vi "subFilterResultsTopLevel.vi"(8 "error in (no error)":errorcluster, 11 "CDependencyInspection in":refnum<class "CDependencyInspection.lvclass">) -> (0 "error out":errorcluster, 3 "CDependencyInspection out":refnum<class "CDependencyInspection.lvclass">)   [LabVIEW 2020, in "DependencyInspection.lvlib" / "CDependencyInspection.lvclass"]
uses:
  CDependencyInspection.lvclass
  CDependencyInspection.lvclass/CDependencyInspection.ctl
  CDependencyList/CDependencyList.lvclass
  obj/Addons/LabVIEWObjectInterfaces.lvlibp/LabVIEWObjectInterfaces/ILabVIEWItem/ILabVIEWItem.lvclass
  obj/Addons/LabVIEWObjectFactory.lvlibp
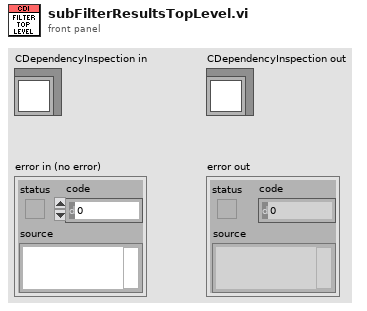
[diagram p1: front panel]
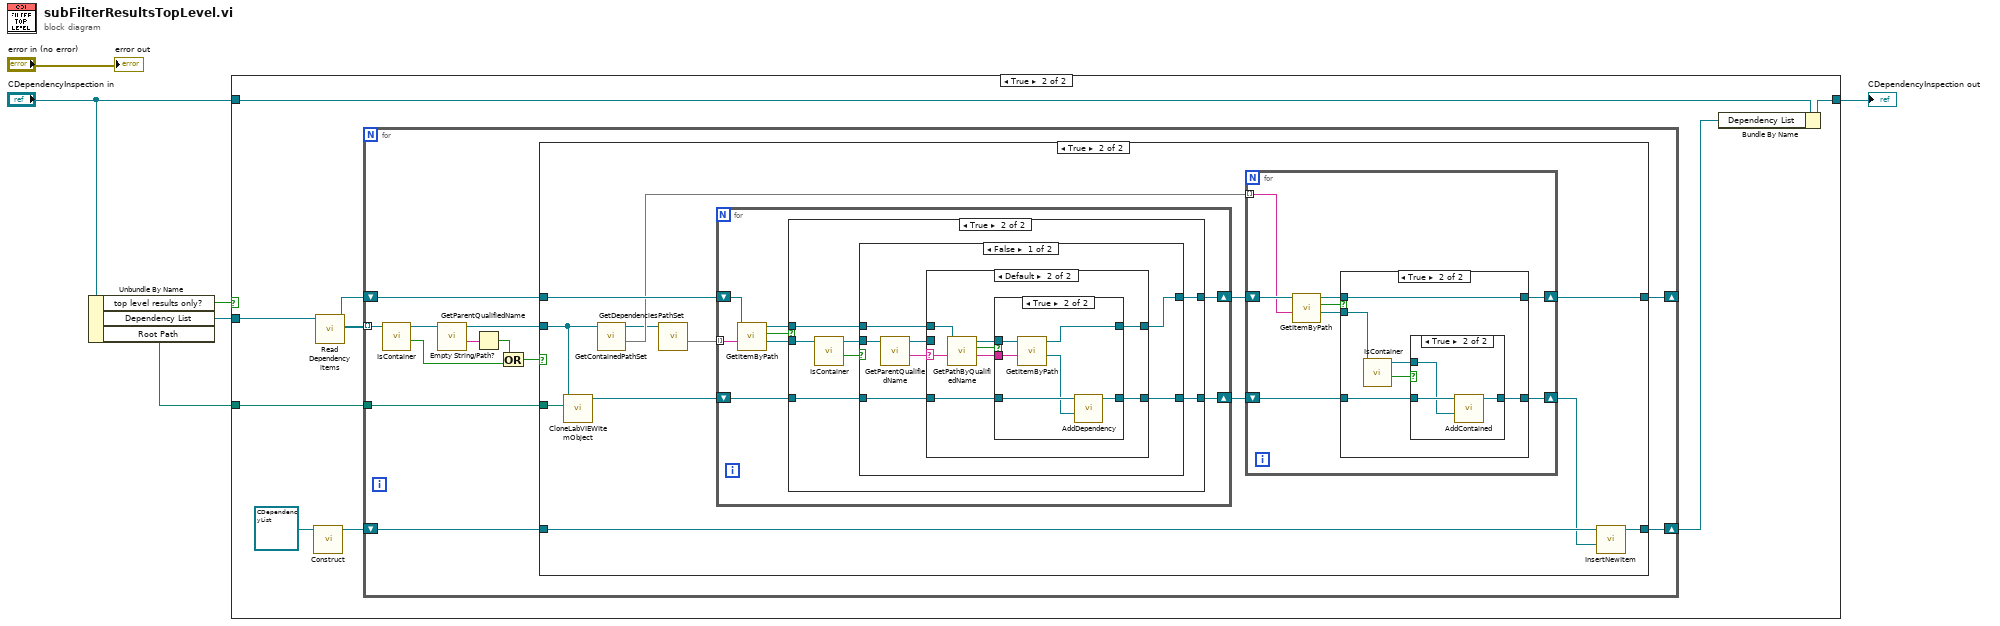
[diagram p0: block diagram]
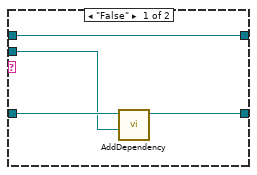
[diagram p5: hidden frame]
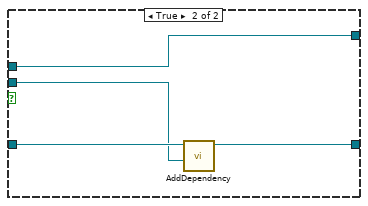
[diagram p7: hidden frame]
diagram:
  n1 = Unbundle By Name("CDependencyInspection in") -> ("top level results only?"=w3:bool, "Dependency List"=w5:refnum<class "CDependencyList.lvclass">, "Root Path"=w4:path)
  n2 = case shown="True" w3 {
    tunnel: w5 -> [_ w13]
    tunnel: w4 -> [_ w12]
    tunnel: "CDependencyInspection in" -> [w7 w10]
    tunnel: [w7 w9] -> w1
    frame False {
    }
    frame True {
      n3 = call-dynamic "Construct.vi"("CDependencyList in"=refnum<class "CDependencyList.lvclass"> refnum) -> ("CDependencyList out"=w11:refnum<class "CDependencyList.lvclass">)  [unwired: 9 in, 1 out]
      n4 = call-dynamic "Read Dependency items.vi"("CDependencyList in"=w13) -> ("Dependency items"=w16:refnum<class "ILabVIEWItem.lvclass">[], "CDependencyList out"=w14:refnum<class "CDependencyList.lvclass">)  [unwired: 9 in]
      n5 = for {
        tunnel: w16 -> [w28] mode=indexing
        shift-right: [w25] -> _
        shift-left: w14 -> [w26]
        tunnel: w12 -> [w27]
        shift-right: [w23] -> w8
        shift-left: w11 -> [w24]
        n6 = call-dynamic "IsContainer.vi"("ILabVIEWItem in"=w28) -> ("Is container?"=w18:bool, "ILabVIEWItem out"=w22:refnum<class "ILabVIEWItem.lvclass">)  [unwired: 8 in, 1 out]
        n7 = call-dynamic "GetParentQualifiedName.vi"("ILabVIEWItem in"=w22) -> ("Name"=w20:string, "ILabVIEWItem out"=w21:refnum<class "ILabVIEWItem.lvclass">)  [unwired: 8 in, 1 out]
        n8 = Empty String/Path?(string/path=w20) -> (empty?=w19:bool)
        n9 = Or(x=w19, y=w18) -> (x .or. y?=w17:bool)
        n10 = case shown="True" w17 {
          tunnel: w27 -> [_ w42]
          tunnel: w26 -> [w30 w40]
          tunnel: [w30 w38] -> w25
          tunnel: w24 -> [w29 w36]
          tunnel: [w29 w34] -> w23
          tunnel: w21 -> [_ w32]
          frame False {
          }
          frame True {
            n11 = call "CloneLabVIEWItemObject.vi"("Root path"=w42, "ILabVIEWItem in"=w32) -> ("Cloned ILabVIEWItem"=w41:refnum<class "ILabVIEWItem.lvclass">)  [unwired: 9 in]
            n12 = call-dynamic "GetContainedPathSet.vi"("ILabVIEWItem in"=w32) -> ("Contained"=w33:set{string}, "ILabVIEWItem out"=w31:refnum<class "ILabVIEWItem.lvclass">)  [unwired: 8 in, 1 out]
            n13 = call-dynamic "GetDependenciesPathSet.vi"("ILabVIEWItem in"=w31) -> ("Dependencies"=w43:set{string})  [unwired: 8 in, 2 out]
            n14 = for {
              tunnel: w43 -> [w51] mode=indexing
              shift-right: [w47] -> w37
              shift-left: w41 -> [w48]
              shift-right: [w44] -> w39
              shift-left: w40 -> [w46]
              n15 = call-dynamic "GetItemByPath.vi"("Path"=w51, "CDependencyList in"=w46) -> ("ILabVIEWItem"=w49:refnum<class "ILabVIEWItem.lvclass">, "key found?"=w50:bool, "CDependencyList out"=w45:refnum<class "CDependencyList.lvclass">)  [unwired: 6 in, 1 out]
              n16 = case shown="True" w50 {
                tunnel: w49 -> [_ w60]
                tunnel: w48 -> [w53 w58]
                tunnel: [w53 w56] -> w47
                tunnel: w45 -> [w52 w55]
                tunnel: [w52 w54] -> w44
                frame False {
                }
                frame True {
                  n17 = call-dynamic "IsContainer.vi"("ILabVIEWItem in"=w60) -> ("Is container?"=w59:bool, "ILabVIEWItem out"=w57:refnum<class "ILabVIEWItem.lvclass">)  [unwired: 8 in, 1 out]
                  n18 = case shown="False" w59 {
                    tunnel: w58 -> [w65 w91]
                    tunnel: w57 -> [w67 w90]
                    tunnel: [w63 w89] -> w56
                    tunnel: w55 -> [w66 w88]
                    tunnel: [w64 w88] -> w54
                    frame False {
                      n19 = call-dynamic "GetParentQualifiedName.vi"("ILabVIEWItem in"=w67) -> ("Name"=w62:string, "ILabVIEWItem out"=w61:refnum<class "ILabVIEWItem.lvclass">)  [unwired: 8 in, 1 out]
                      n20 = case shown="Default" w62 {
                        selector: w62 -> [_ w72]
                        tunnel: w66 -> [w68 w79]
                        tunnel: w65 -> [w71 w75]
                        tunnel: [w68 w74] -> w64
                        tunnel: [w70 w73] -> w63
                        tunnel: w61 -> [w69 _]
                        frame "False" {
                          n21 = call-dynamic "AddDependency.vi"("Item to depend on"=w69, "ILabVIEWItem in"=w71) -> ("ILabVIEWItem out"=w70:refnum<class "ILabVIEWItem.lvclass">)  [unwired: 8 in, 1 out]
                        }
                        frame Default {
                          n22 = call-dynamic "GetPathByQualifiedName.vi"("Qualified name"=w72, "CDependencyList in"=w79) -> ("Path"=w77:string, "key found?"=w78:bool, "CDependencyList out"=w76:refnum<class "CDependencyList.lvclass">)  [unwired: 6 in, 1 out]
                          n23 = case shown="True" w78 {
                            tunnel: w77 -> [_ w86]
                            tunnel: w76 -> [w81 w87]
                            tunnel: w75 -> [w80 w85]
                            tunnel: [w81 w83] -> w74
                            tunnel: [w80 w82] -> w73
                            frame False {
                            }
                            frame True {
                              n24 = call-dynamic "GetItemByPath.vi"("Path"=w86, "CDependencyList in"=w87) -> ("ILabVIEWItem"=w84:refnum<class "ILabVIEWItem.lvclass">, "CDependencyList out"=w83:refnum<class "CDependencyList.lvclass">)  [unwired: 6 in, 2 out]
                              n25 = call-dynamic "AddDependency.vi"("Item to depend on"=w84, "ILabVIEWItem in"=w85) -> ("ILabVIEWItem out"=w82:refnum<class "ILabVIEWItem.lvclass">)  [unwired: 8 in, 1 out]
                            }
                          }
                        }
                      }
                    }
                    frame True {
                      n26 = call-dynamic "AddDependency.vi"("Item to depend on"=w90, "ILabVIEWItem in"=w91) -> ("ILabVIEWItem out"=w89:refnum<class "ILabVIEWItem.lvclass">)  [unwired: 8 in, 1 out]
                    }
                  }
                }
              }
            }
            n27 = for {
              tunnel: w33 -> [w98] mode=indexing
              shift-right: [w93] -> w38
              shift-left: w39 -> [w99]
              shift-right: [w94] -> w35
              shift-left: w37 -> [w95]
              n28 = call-dynamic "GetItemByPath.vi"("Path"=w98, "CDependencyList in"=w99) -> ("ILabVIEWItem"=w96:refnum<class "ILabVIEWItem.lvclass">, "key found?"=w97:bool, "CDependencyList out"=w92:refnum<class "CDependencyList.lvclass">)  [unwired: 6 in, 1 out]
              n29 = case shown="True" w97 {
                tunnel: w96 -> [_ w107]
                tunnel: w95 -> [w101 w104]
                tunnel: [w101 w103] -> w94
                tunnel: [w100 w102] -> w93
                tunnel: w92 -> [w100 w102]
                frame False {
                }
                frame True {
                  n30 = call-dynamic "IsContainer.vi"("ILabVIEWItem in"=w107) -> ("Is container?"=w105:bool, "ILabVIEWItem out"=w106:refnum<class "ILabVIEWItem.lvclass">)  [unwired: 8 in, 1 out]
                  n31 = case shown="True" w105 {
                    tunnel: w106 -> [_ w110]
                    tunnel: w104 -> [w108 w111]
                    tunnel: [w108 w109] -> w103
                    frame False {
                    }
                    frame True {
                      n32 = call-dynamic "AddContained.vi"("Item to contain"=w110, "ILabVIEWItem in"=w111) -> ("ILabVIEWItem out"=w109:refnum<class "ILabVIEWItem.lvclass">)  [unwired: 8 in, 1 out]
                    }
                  }
                }
              }
            }
            n33 = call-dynamic "InsertNewItem.vi"("ILabVIEWItem in"=w35, "CDependencyList in"=w36) -> ("CDependencyList out"=w34:refnum<class "CDependencyList.lvclass">)  [unwired: 7 in, 2 out]
          }
        }
      }
      n34 = Bundle By Name(cluster=w10, "Dependency List"=w8) -> (w9:refnum<class "CDependencyInspection.lvclass">)
    }
  }
  "CDependencyInspection out" <- w1
  "error out" <- "error in (no error)"
